vi "Move_Nanostage.vi"(0 "position":dbl[](array[numeric]), 1 "Down":bool, 2 "^":bool, 3 "v":bool, 4 "keys pressed":T1(array[ring]), 5 "error in (no error)":errorcluster, 7 "<":bool, 9 ">":bool, 10 "handle in":i32, 11 "Up":bool, 12 "step size":dbl) -> (14 "handle out":i32, 19 "error out":errorcluster)   [LabVIEW 2019]
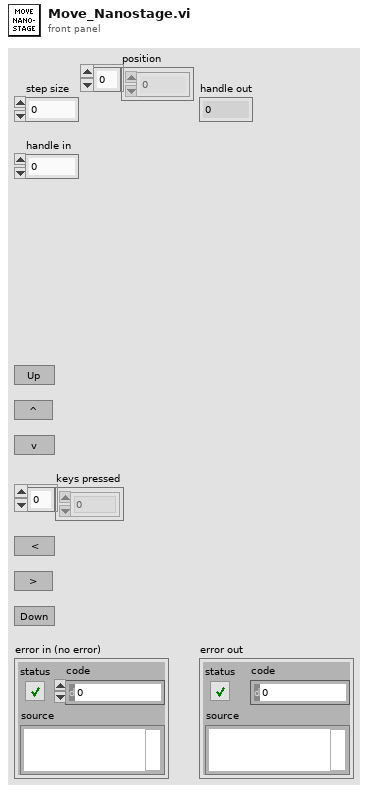
[diagram p1: front panel]
types:
  T1 = enum16{"0", "1", "2", "3", "4", "5", "6", "7", "8", "9", "A", "B", "C", "D", "E", "F", "G", "H", "I", "J", "K", "L", "M", "N", "O", "P", "Q", "R", "S", "T", "U", "V", "W", "X", "Y", "Z", "F1", "F2", "F3", "F4", "F5", "F6", "F7", "F8", "F9", "F10", "F11", "F12", "F13", "F14", "F15", "ADD", "BACK", "BACKSLASH", "CAPITAL", "COMMA", "DECIMAL", "DELETE", "DIVIDE", "DOWN", "END", "EQUALS", "ESCAPE", "GRAVE (`)", "HOME", "INSERT", "LBRACKET", "LCONTROL", "LEFT", "L ALT", "LSHIFT", "LWIN", "MINUS", "MULTIPLY", "NEXT", "NUMLOCK", "NUMPAD_0", "NUMPAD_1", "NUMPAD_2", "NUMPAD_3", "NUMPAD_4", "NUMPAD_5", "NUMPAD_6", "NUMPAD_7", "NUMPAD_8", "NUMPAD_9", "PAUSE", "PERIOD", "PRIOR (PG UP)", "RBRACKET", "RCONTROL", "RETURN", "RIGHT", "R ALT", "RSHIFT", "RWIN", "SCROLL", "SEMICOLON", "SLASH", "SPACE", "SUBTRACT", "TAB", "UP", "ENTER (num pad)", "' (quote)"}[]
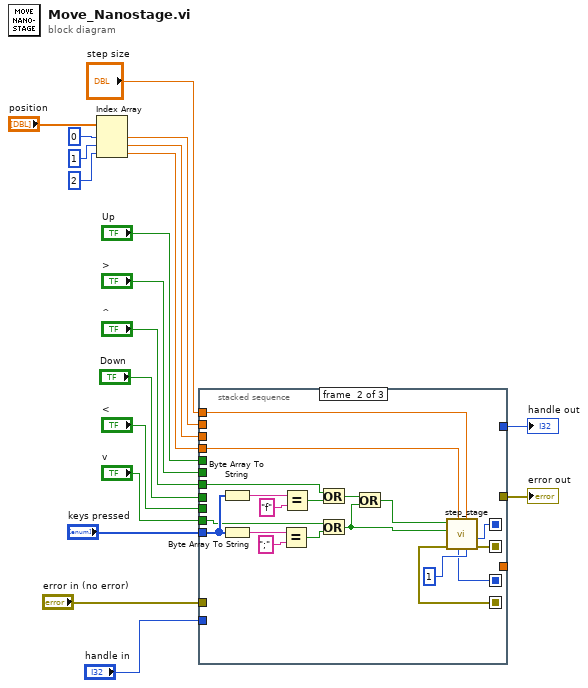
[diagram p0: block diagram]
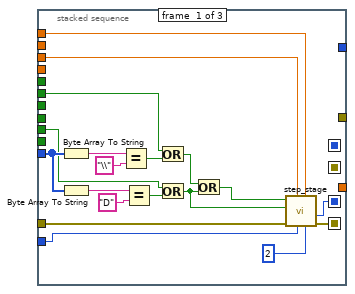
[diagram p2: hidden frame]
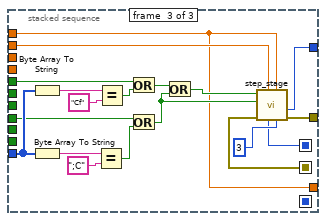
[diagram p3: hidden frame]
diagram:
  n1 = Index Array(array="position", index #1=0 ("index"), index #2=1 ("index"), index #3=2 ("index")) -> (element #1=w7:dbl, element #2=w5:dbl, element #3=w4:dbl)
  n2 = stacked-sequence {
    seq-local: [w34 _ _] -> [_ w54 _]
    seq-local: [w33 _ _] -> [_ w53 _]
    seq-local: [_ w51 _] -> [_ _ w72]
    seq-local: [_ w52 _] -> [_ _ w71]
    tunnel: "error in (no error)" -> [w38 _ _]
    tunnel: "handle in" -> [w37 _ _]
    tunnel: w5 -> [w35 _ _]
    tunnel: w4 -> [_ w55 _]
    tunnel: w7 -> [_ _ w75]
    tunnel: [_ _ w73] -> w12
    tunnel: [_ _ w74] -> w11
    tunnel: "keys pressed" -> [w23 w42 w61]
    tunnel: [_ _ w60] -> _
    tunnel: "step size" -> [w22 w41 w60]
    tunnel: "Down" -> [_ _ w59]
    tunnel: "Up" -> [_ _ w58]
    tunnel: "<" -> [w21 _ _]
    tunnel: ">" -> [w20 _ _]
    tunnel: "^" -> [_ w40 _]
    tunnel: "v" -> [_ w39 _]
    frame #0 {
      n3 = Byte Array To String(unsigned byte array=w23) -> (string=w32:string)
      n4 = Byte Array To String(unsigned byte array=w23) -> (string=w30:string)
      n5 = Equal?(x=w32, y="\\") -> (x = y?=w28:bool)
      n6 = Equal?(x=w30, y="D") -> (x = y?=w27:bool)
      n7 = Or(x=w20, y=w28) -> (x .or. y?=w26:bool)
      n8 = Or(x=w21, y=w27) -> (x .or. y?=w25:bool)
      n9 = Or(x=w26, y=w25) -> (x .or. y?=w24:bool)
      n10 = call "step_stage.vi"("axis"=u32 2, "step"=w22, "handle"=w37, "position"=w35, "error in"=w38, "+/-"=w25, "move"=w24) -> ("error out"=w33:errorcluster, "handle out"=w34:i32)  [unwired: 3 in]
    }
    frame #1 {
      n11 = Byte Array To String(unsigned byte array=w42) -> (string=w50:string)
      n12 = Byte Array To String(unsigned byte array=w42) -> (string=w48:string)
      n13 = Equal?(x=w48, y=";") -> (x = y?=w45:bool)
      n14 = Equal?(x=w50, y="f") -> (x = y?=w46:bool)
      n15 = Or(x=w40, y=w46) -> (x .or. y?=w44:bool)
      n16 = Or(x=w39, y=w45) -> (x .or. y?=w43:bool)
      n17 = Or(x=w44, y=w43) -> (x .or. y?=w57:bool)
      n18 = call "step_stage.vi"("axis"=u32 1, "step"=w41, "handle"=w54, "position"=w55, "error in"=w53, "+/-"=w43, "move"=w57) -> ("error out"=w52:errorcluster, "handle out"=w51:i32)  [unwired: 3 in]
    }
    frame #2 {
      n19 = Byte Array To String(unsigned byte array=w61) -> (string=w70:string)
      n20 = Byte Array To String(unsigned byte array=w61) -> (string=w68:string)
      n21 = Equal?(x=w68, y=";C") -> (x = y?=w65:bool)
      n22 = Equal?(x=w70, y="Cf") -> (x = y?=w66:bool)
      n23 = Or(x=w58, y=w66) -> (x .or. y?=w64:bool)
      n24 = Or(x=w59, y=w65) -> (x .or. y?=w62:bool)
      n25 = Or(x=w64, y=w62) -> (x .or. y?=w63:bool)
      n26 = call "step_stage.vi"("axis"=u32 3, "step"=w60, "handle"=w72, "position"=w75, "error in"=w71, "+/-"=w62, "move"=w63) -> ("error out"=w73:errorcluster, "handle out"=w74:i32)  [unwired: 3 in]
    }
  }
  "error out" <- w12
  "handle out" <- w11
